vi "ArmInvalidateHomePositions.vi"(4 "ArmHomingValidityIn":T2=enum."Invalid", 5 "ArmPositionValidityIn":T4, 6 "ArmHomingStateIn":T3=enum."homing failed", 7 "ArmRecoveryParameters In":T1) -> (0 "ArmHomingValidityOut":T2=enum."Invalid", 1 "ArmPositionValidityOut":T4, 2 "ArmHomingStateOut":T3=enum."homing failed", 3 "ArmRecoveryParameters Out":T1)   [LabVIEW 2018]
uses:
  TypeDefs/ArmPositionComponentValidity.ctl
  TypeDefs/ArmPositionRecoveryParams.ctl
  TypeDefs/ArmHomingState.ctl
  TypeDefs/ArmHomingValidity.ctl
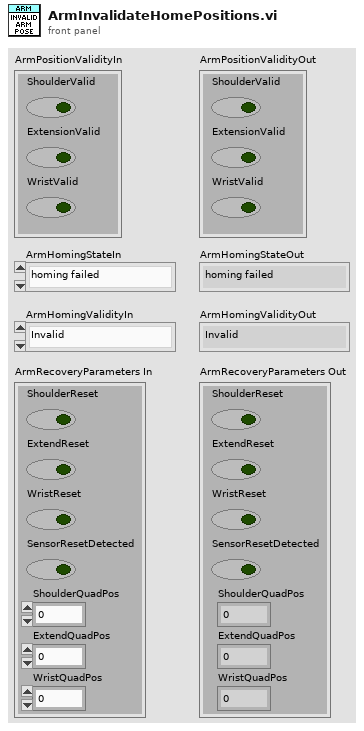
[diagram p1: front panel]
types:
  T1 = typedef "ArmPositionRecoveryParams.ctl" = cluster{"ShoulderReset":bool, "ExtendReset":bool, "WristReset":bool, "SensorResetDetected":bool, "ShoulderQuadPos":i32, "ExtendQuadPos":i32, "WristQuadPos":i32}
  T2 = typedef "ArmHomingValidity.ctl" = enum16{"Incomplete", "Valid", "Invalid"}
  T3 = typedef "ArmHomingState.ctl" = enum16{"ready", "homing in progress", "homing complete ", "homing failed"}
  T4 = typedef "ArmPositionComponentValidity.ctl" = cluster{"ShoulderValid":bool, "ExtensionValid":bool, "WristValid":bool}
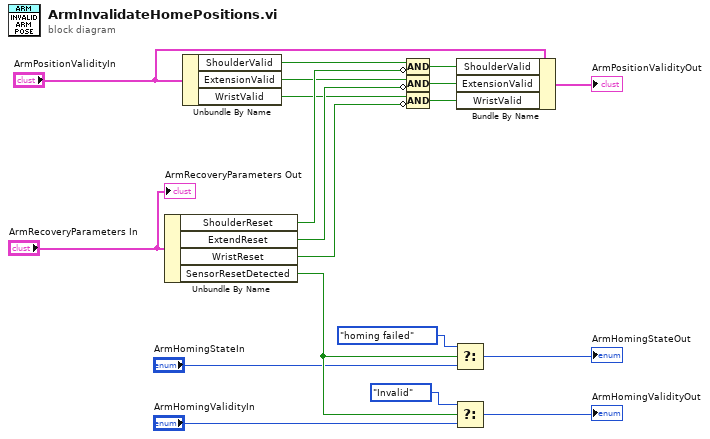
[diagram p0: block diagram]
diagram:
  n1 = Unbundle By Name("ArmRecoveryParameters In") -> ("ShoulderReset"=w18:bool, "ExtendReset"=w16:bool, "WristReset"=w14:bool, "SensorResetDetected"=w8:bool)
  n2 = Unbundle By Name("ArmPositionValidityIn") -> ("ShoulderValid"=w19:bool, "ExtensionValid"=w17:bool, "WristValid"=w15:bool)
  n3 = Compound Arithmetic op=AND(w19, invert w18) -> (w12:bool)
  n4 = Compound Arithmetic op=AND(w17, invert w16) -> (w11:bool)
  n5 = Compound Arithmetic op=AND(w15, invert w14) -> (w10:bool)
  n6 = Select(t=ArmHomingState."homing failed" ("arm homing state"), s=w8, f="ArmHomingStateIn") -> (s? t:f=→"ArmHomingStateOut":T3)
  n7 = Select(t=ArmHomingValidity."Invalid" ("arm homing validity"), s=w8, f="ArmHomingValidityIn") -> (s? t:f=→"ArmHomingValidityOut":T2)
  n8 = Bundle By Name(cluster="ArmPositionValidityIn", "ShoulderValid"=w12, "ExtensionValid"=w11, "WristValid"=w10) -> (→"ArmPositionValidityOut":T4)
  "ArmRecoveryParameters Out" <- "ArmRecoveryParameters In"
